vi "Pre-Actor.vi"(8 "error in":errorcluster, 11 "SwitchMatrix in":refnum<class "SwitchMatrix.lvclass">) -> (0 "error out":errorcluster, 3 "SwitchMatrix out":refnum<class "SwitchMatrix.lvclass">)   [LabVIEW 2019, in "SwitchMatrix.lvlib" / "SwitchMatrix.lvclass"]
doc: "This override VI is to provide the means for children classes to perform application specific post launch initialization functions that must be performed *prior* to calling the actor. \n\n***DO NOT USE THE CHECK FOR FAULT ROUTINE HERE***"
uses:
  Library/SwitchMatrix.lvclass
  builds/Instruments/Instruments.lvlibp/Library/Instruments.lvclass
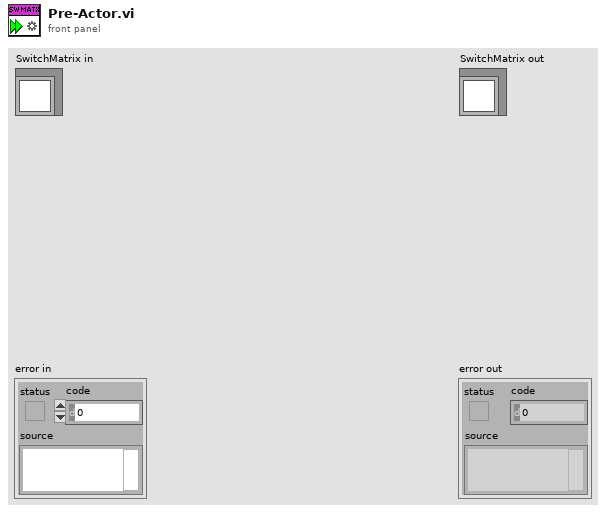
[diagram p1: front panel]
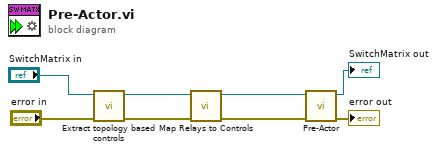
[diagram p0: block diagram]
diagram:
  n1 = call "Extract topology based controls.vi"("error in"="error in", "SwitchMatrix in"="SwitchMatrix in") -> ("error out"=w3:errorcluster, "SwitchMatrix out"=w4:refnum<class "SwitchMatrix.lvclass">)  [unwired: 8 in]
  n2 = call "Map Relays to Controls.vi"("error in (no error)"=w3, "SwitchMatrix in"=w4) -> ("error out"=w1:errorcluster, "SwitchMatrix out"=w2:refnum<class "SwitchMatrix.lvclass">)  [unwired: 8 in]
  n3 = call-parent "Pre-Actor.vi"("error in (no error)"=w1, "Instruments in"=w2) -> ("error out"=→"error out":errorcluster, "Instruments out"=→"SwitchMatrix out":refnum<class "SwitchMatrix.lvclass">)  [unwired: 8 in]
